vi "Valid.vi"(11 "QueueMessenger in":refnum<class "QueueMessenger.lvclass">) -> (2 "Valid?":bool, 3 "QueueMessenger out":refnum<class "QueueMessenger.lvclass">)   [LabVIEW 2011, in "Messenging.lvlib" / "QueueMessenger.lvclass"]
uses:
  QueueMessenger.lvclass
  QueueMessenger.lvclass/QueueMessenger.ctl
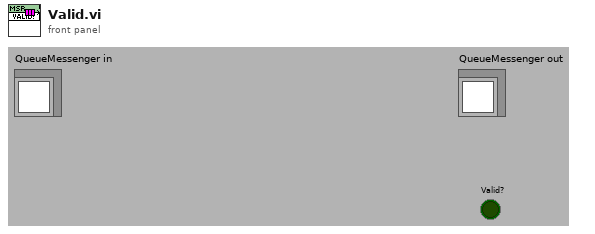
[diagram p1: front panel]
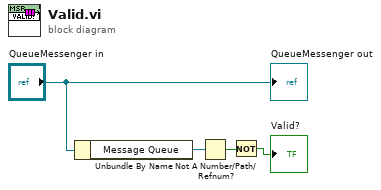
[diagram p0: block diagram]
diagram:
  n1 = Unbundle By Name("QueueMessenger in") -> ("Message Queue"=w4:refnum<queue>)
  n2 = Not A Number/Path/Refnum?(number/path/refnum=w4) -> (NaN/Path/Refnum?=w3:bool)
  n3 = Not(x=w3) -> (.not. x?=→"Valid?":bool)
  "QueueMessenger out" <- "QueueMessenger in"
